vi "event_channel.vi"() -> ()   [LabVIEW 2021]
uses:
  <extravilib>/ChannelInstances/Event Messenger-dbl/Instantiate.vi
  <extravilib>/ChannelInstances/Event Messenger-dbl/))Channel.vi
  <extravilib>/ChannelInstances/Event Messenger-dbl.lvlib
panel:
  out "Waveform Chart":dbl(graph)
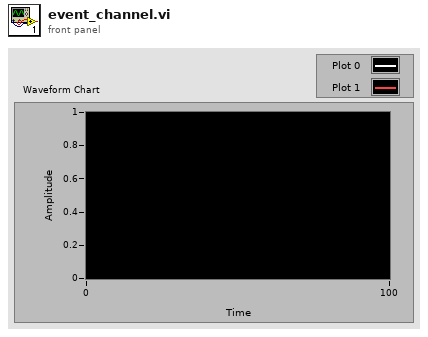
[diagram p1: front panel]
types:
  T1 = typedef "Event Messenger-dbl.lvlib/))Channel.ctl" = refnum<queue>
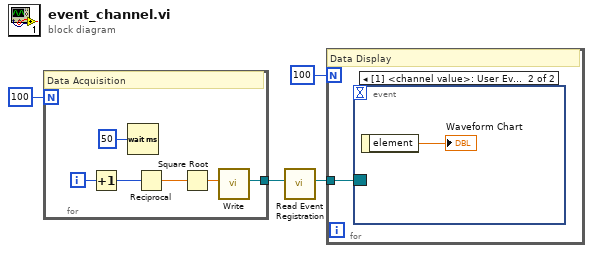
[diagram p0: block diagram]
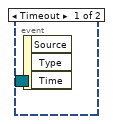
[diagram p2: hidden frame]
diagram:
  n1 = for {
    N: 100 -> [_]
    tunnel: [w7] -> w2
    i -> [w9]
    # "Data Acquisition"
    n2 = Increment(x=w9) -> (x+1=w8:i32)
    n3 = Wait (ms)(milliseconds to wait=u32 50) -> ()  [unwired: 1 out]
    n4 = Reciprocal(x=w8) -> (1/x=w6:dbl)
    n5 = Square Root(x=w6) -> (sqrt(x)=w5:dbl)
    n6 = call <extravilib>:"Write.vi"("element"=w5) -> ("channel"=w7:T1)  [unwired: 9 in, 1 out]
  }
  n7 = call <extravilib>:"Read Event Registration.vi"("channel"=w2) -> ("event registration refnum"=w1:refnum<event-registration>)  [unwired: 10 in]
  n8 = for {
    N: 100 -> [_]
    tunnel: w1 -> [w11]
    # "Data Display"
    n9 = event shown="[1] <channel value>: User Event" {
      selector: w11 -> [_ _]
      dyn-events: _ -> [_ _]
      timeout: _ -> [_ _]
      event Timeout {
        n10 = event-data() -> ()  [unwired: 1 in, 3 out]
      }
      event User Event {
        n11 = event-data() -> ("element"=→"Waveform Chart":dbl)  [unwired: 1 in]
      }
    }
  }
